vi "CtrlRefProbe.vi"(11 "Control Refnum":refnum<vi>) -> (2 "Display string":string, 3 "Pause VI":bool)   [LabVIEW 2020]
doc: "Displays the class name, the control label, the hex value of the reference, the VI name of the owner, and the path of the VI. You can use this probe to pause if the value is an invalid refnum."
uses:
  <vilib>/Utility/error.llb/DialogTypeEnum.ctl
panel:
  in  "owning VI":string="Owning VI"
  in  "control label":string="Control label"
  in  "class name":string="Class name"
  in  "error source":string="Control Refnum Probe"
  in  "Pause if Not a Refnum":bool
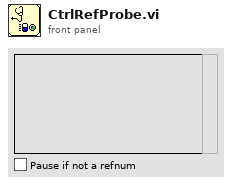
[diagram p1: front panel]
types:
  T1 = typedef "DialogTypeEnum.ctl" = enum16{"no dialog", "OK message", "continue or stop message", "auto error handling dialog", "OK message + warnings", "continue/stop + warnings"}
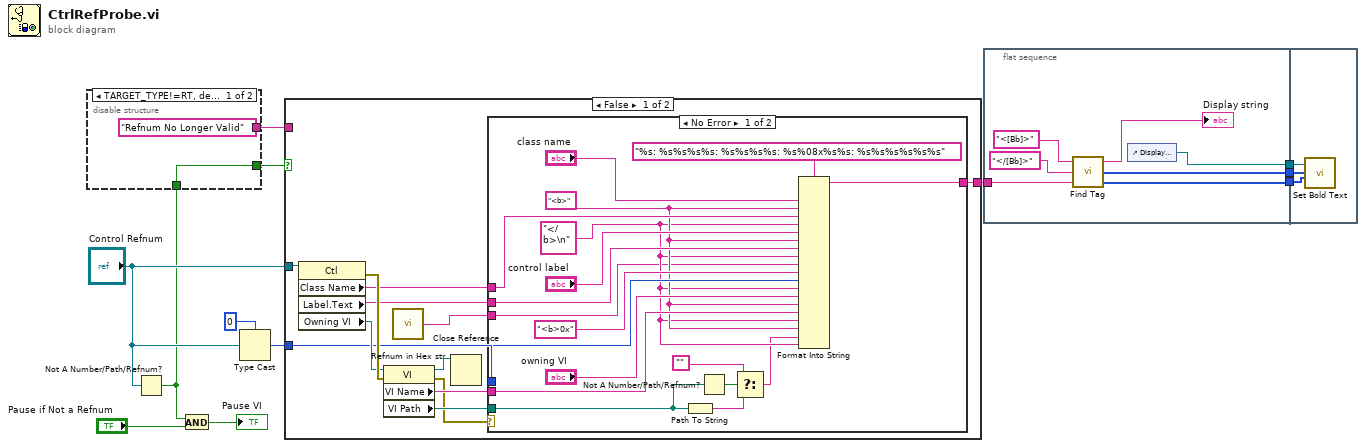
[diagram p0: block diagram]
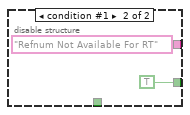
[diagram p2: hidden frame]
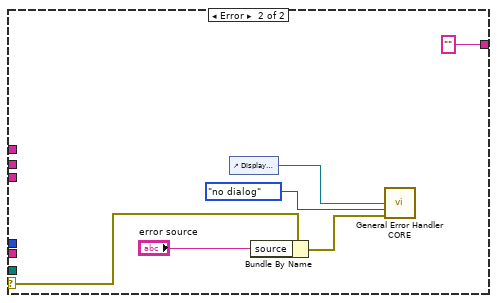
[diagram p3: hidden frame]
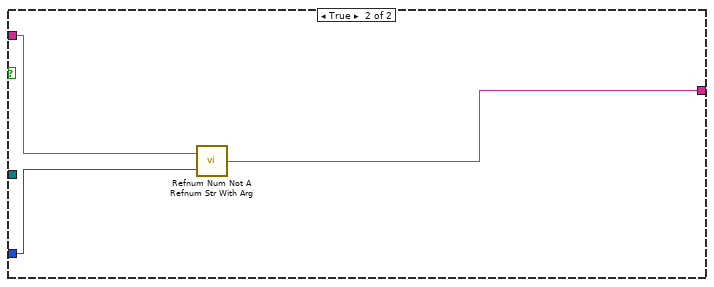
[diagram p4: hidden frame]
diagram:
  n1 = Not A Number/Path/Refnum?(number/path/refnum="Control Refnum") -> (NaN/Path/Refnum?=w6:bool)
  n2 = disable-structure shown="TARGET_TYPE!=RT, default" {
    disable-tunnel: ["Refnum No Longer Valid" "Refnum Not Available For RT"] -> w7
    disable-tunnel: w6 -> [w13 _]
    disable-tunnel: [w13 TRUE] -> w5
    frame condition #0 (active) {
    }
    frame condition #1 {
    }
  }
  n3 = And(x=w6, y="Pause if Not a Refnum") -> (x .and. y?=→"Pause VI":bool)
  n4 = Type Cast(type=u32 0, x="Control Refnum") -> (*(type *) &x=w8:u32)
  n5 = case shown="False" w5 {
    tunnel: "Control Refnum" -> [w22 _]
    tunnel: w8 -> [w19 w54]
    tunnel: w7 -> [_ w55]
    tunnel: [w17 w53] -> w4
    frame False {
      n6 = property class="Ctl"(reference=w22) -> (error out=w28:errorcluster, "Class Name"=w26:string, "Label.Text"=w25:string, "Owning VI"=w27:refnum<vi>)  [unwired: 1 in, 1 out]
      n7 = property class="VI"(reference=w27, error in=w28) -> (reference out=w20:refnum<vi>, error out=w21:errorcluster, "VI Name"=w24:string, "VI Path"=w23:path)
      n8 = call <vilib>:"Refnum in Hex str.vi"() -> ("refnum in hex"=w18:string)
      n9 = Close Reference(reference=w20) -> ()  [unwired: 1 in, 1 out]
      n10 = case shown="No Error" w21 {
        selector: w21 -> [_ w50]
        tunnel: w26 -> [w45 _]
        tunnel: w25 -> [w43 _]
        tunnel: w19 -> [w41 _]
        tunnel: w24 -> [w39 _]
        tunnel: w23 -> [w34 _]
        tunnel: w18 -> [w30 _]
        tunnel: [w29 ""] -> w17
        frame No Error {
          w37 = "</b>\n"
          w38 = "<b>"
          n11 = Path To String(path=w34) -> (string=w33:string)
          n12 = Not A Number/Path/Refnum?(number/path/refnum=w34) -> (NaN/Path/Refnum?=w35:bool)
          n13 = Select(t="", s=w35, f=w33) -> (s? t:f=w31:string)
          n14 = Format Into String(format string="%s: %s%s%s%s: %s%s%s%s: %s%08x%s%s: %s%s%s%s%s%s", "class name", w38, w45, w37, "control label", w38, w43, w37, w30, "<b>0x", w41, w37, "owning VI", w38, w39, w37, w38, w31, w37) -> (resulting string=w29:string)  [unwired: 2 in, 1 out]
        }
        frame Error {
          n15 = control-ref of="Display string"() -> (w51:refnum<vi>)
          n16 = Bundle By Name(cluster=w50, "source"="error source") -> (w48:errorcluster)
          n17 = call <vilib>:"General Error Handler CORE.vi"("String to Format (not a refnum)"=w51, "type of dialog (OK msg:1)"=DialogTypeEnum."no dialog", "error in (no error)"=w48) -> ()  [unwired: 7 in, 6 out]
        }
      }
    }
    frame True {
      n18 = call <vilib>:"Refnum Num Not A Refnum Str With Arg.vi"("Numeric"=w54, "failure message"=w55) -> ("text to display"=w53:string)
    }
  }
  n19 = flat-sequence {
    tunnel: w4 -> [w60]
    tunnel: [w58] -> w3
    tunnel: [w57] -> w2
    tunnel: [w56] -> w1
    tunnel: w3 -> [w65]
    tunnel: w2 -> [w64]
    tunnel: w1 -> [w63]
    frame #0 {
      n20 = call <vilib>:"Find Tag.vi"("string"=w60, "close tag"="</[Bb]>", "open tag"="<[Bb]>") -> ("Length"=w58:i32[], "Start"=w57:i32[], "string out"=→"Display string":string)
      n21 = control-ref of="Display string"() -> (w56:refnum<vi>)
    }
    frame #1 {
      n22 = call <vilib>:"Set Bold Text.vi"("Length"=w65, "Start"=w64, "text"=w63) -> ()  [unwired: 3 in, 1 out]
    }
  }
